vi "PipBoy_InitMain.vi"(8 "error in (no error)":errorcluster) -> (0 "error out":errorcluster, 2 "PipBoyData":T2, 3 "DynamicUE":T1)   [LabVIEW 2014]
uses:
  ctls/PipBoy_PipBoyData.ctl
  ctls/PipBoy_ProcComm.ctl
  System.Windows.Forms
  ctls/PipBoy_PipBoyCommand.ctl
  ctls/PipBoy_Message.ctl
  modules/support/Message Queue/All Message Queues.ctl
  modules/support/Message Queue/Message Cluster.ctl
  ctls/PipBoy_FileConf.ctl
  ctls/PipBoy_PicComm.ctl
  ctls/PipBoy_GeneralParams.ctl
  ctls/PipBoy_Pages.ctl
  <userlib>/NotifyIcon/TypeDefs/NotifyIcon User Event Ref.ctl
  modules/support/User Event - Stop/User Event - Stop.lvlib
  modules/support/Message Queue/Message Queue.lvlib
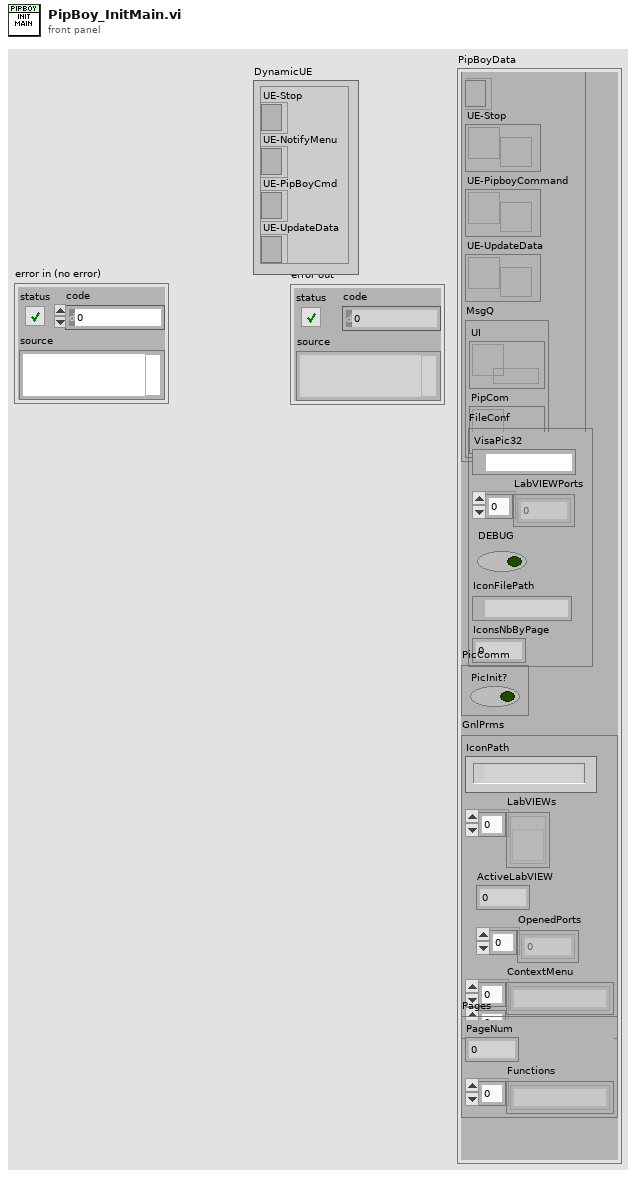
[diagram p1: front panel]
types:
  T1 = cluster{"UE-Stop":refnum<event-registration>, "UE-NotifyMenu":refnum<event-registration>, "UE-PipBoyCmd":refnum<event-registration>, "UE-UpdateData":refnum<event-registration>}
  T2 = typedef "PipBoy_PipBoyData.ctl" = cluster{"ProcComm":T3, "FileConf":T5, "PicComm":T6, "GnlPrms":T7, "Pages":T8}
  T3 = typedef "PipBoy_ProcComm.ctl" = cluster{"NotifyIconRef":refnum<k24>, "UE-Stop":refnum<user-event>, "UE-PipboyCommand":refnum<user-event>, "UE-UpdateData":refnum<user-event>, "MsgQ":T4}
  T4 = typedef "Message Queue.lvlib/All Message Queues.ctl" = cluster{"UI":refnum<queue>, "PipCom":refnum<queue>}
  T5 = typedef "PipBoy_FileConf.ctl" = cluster{"VisaPic32":refnum<visa-resource-name>, "LabVIEWPorts":u16[], "DEBUG":bool, "IconFilePath":path, "IconsNbByPage":i32}
  T6 = typedef "PipBoy_PicComm.ctl" = cluster{"PicInit?":bool}
  T7 = typedef "PipBoy_GeneralParams.ctl" = cluster{"IconPath":path, "LabVIEWs":refnum<vi>[], "ActiveLabVIEW":i32, "OpenedPorts":u16[], "ContextMenu":string[][]}
  T8 = typedef "PipBoy_Pages.ctl" = cluster{"PageNum":i32, "Functions":string[]}
  T9 = cluster{"Stop Event Registration Refnum":refnum<event-registration>, "UE-NotifyMenu":refnum<event-registration>, "UE-PipBoyCmd":refnum<event-registration>, "UE-UpdateData":refnum<event-registration>}
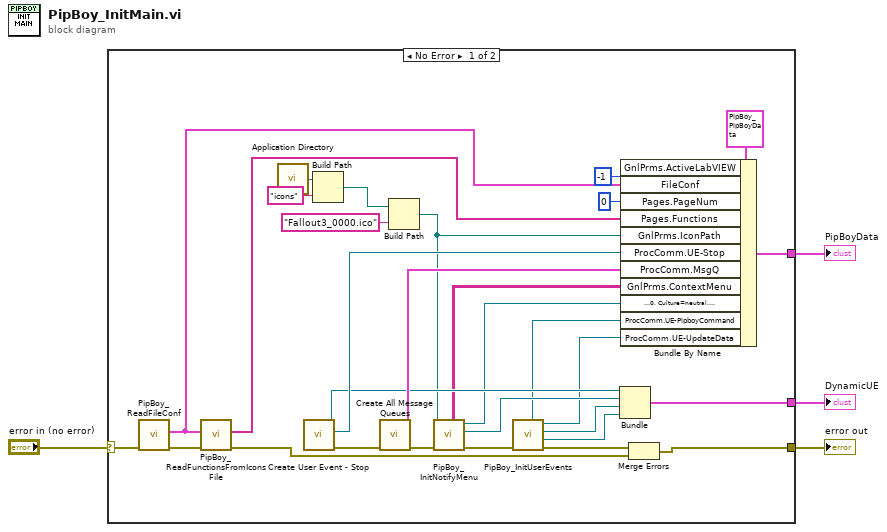
[diagram p0: block diagram]
diagram:
  n1 = case shown="No Error" "error in (no error)" {
    selector: "error in (no error)" -> [w21 w35]
    tunnel: [w19 w35] -> w3
    tunnel: [w30 _] -> w2
    tunnel: [w29 _] -> w1
    frame No Error {
      n2 = call "PipBoy_ReadFileConf.vi"("error in (no error)"=w21) -> ("error out"=w13:errorcluster, "FileConf"=w11:T5)  [unwired: 9 in]
      n3 = call "PipBoy_ReadFunctionsFromIconsFile.vi"("error in (no error)"=w13, "FileConf"=w11) -> ("error out"=w12:errorcluster, "Functions"=w9:string[])  [unwired: 8 in]
      n4 = call <vilib>:"Application Directory.vi"() -> ("Application Directory"=w25:path)
      n5 = call "Create User Event - Stop.vi"() -> ("error out"=w34:errorcluster, "User Event - Stop"=w31:refnum<user-event>, "Stop Event Registration Refnum"=w28:refnum<event-registration>)  [unwired: 9 in]
      n6 = Build Path(base path=w25, name or relative path="icons") -> (appended path=w23:path)
      n7 = call "Create All Message Queues.vi"("error in (no error)"=w34) -> ("error out"=w26:errorcluster, "Message Queues out"=w32:T4)  [unwired: 9 in]
      n8 = Build Path(base path=w23, name or relative path="Fallout3_0000.ico") -> (appended path=w20:path)
      n9 = call "PipBoy_InitNotifyMenu.vi"("error in (no error)"=w26, "IconPath"=w20) -> ("error out"=w16:errorcluster, "UE-NotifyMenu"=w27:refnum<event-registration>, "NotifyIconRef"=w18:refnum<k24>, "Context Menu"=w17:string[][])  [unwired: 6 in]
      n10 = call "PipBoy_InitUserEvents.vi"("error in (no error)"=w16) -> ("error out"=w15:errorcluster, 1:"UE-UpdateData"=w5:refnum<event-registration>, "UE-PipBoyCmd"=w6:refnum<event-registration>, 3:"UE-UpdateData"=w7:refnum<user-event>, "UE-PipboyCommand"=w8:refnum<user-event>)  [unwired: 6 in]
      n11 = Bundle("Stop Event Registration Refnum"=w28, "UE-NotifyMenu"=w27, "UE-PipBoyCmd"=w6, "UE-UpdateData"=w5) -> (w29:T9)  [unwired: 1 in]
      n12 = Bundle By Name(cluster=T2 {"ProcComm"={"NotifyIconRef"=refnum, "UE-Stop"=refnum, "UE-PipboyCommand"=refnum, "UE-UpdateData"=refnum, "MsgQ"={"UI"=refnum, "PipCom"=refnum}}, "FileConf"={"VisaPic32"="", "LabVIEWPorts"=[], "DEBUG"=FALSE, "IconFilePath"=path "", "IconsNbByPage"=0}, "PicComm"={"PicInit?"=FALSE}, "GnlPrms"={"IconPath"=path "", "LabVIEWs"=[], "ActiveLabVIEW"=0, "OpenedPorts"=[], "ContextMenu"=[]}, "Pages"={"PageNum"=0, "Functions"=[]}} ("input cluster"), "GnlPrms.ActiveLabVIEW"=-1, "FileConf"=w11, "Pages.PageNum"=0 ("Pages.PageNb"), "Pages.Functions"=w9, "GnlPrms.IconPath"=w20, "ProcComm.UE-Stop"=w31, "ProcComm.MsgQ"=w32, "GnlPrms.ContextMenu"=w17, "ProcComm.NotifyIconRef"=w18, "ProcComm.UE-PipboyCommand"=w8, "ProcComm.UE-UpdateData"=w7) -> (w30:T2)
      n13 = Merge Errors(w15, w12) -> (w19:errorcluster)
    }
    frame Error {
    }
  }
  "error out" <- w3
  "PipBoyData" <- w2
  "DynamicUE" <- w1
